vi "New Image (ARGB Array).vi"(7 "Set Alpha Values to 255 (Default: True)":bool=TRUE, 8 "error in (no error)":errorcluster, 11 "U32 ARBG Data":u32[][](array[numeric])) -> (0 "error out":errorcluster, 3 "ARGB Image":T1)   [LabVIEW 2020, in "image.lvlib"]
doc: "Create a New Image. The New Image data can be prep-populated with the given array of U32 image data.\n\nTo create a New Image which has a preallocated size with a uniform colour, use the \"New Image (ARGB Preallocated).vi\""
uses:
  image.lvlib
  ARGB Image.ctl
  common/common.lvlib
  common/bin/gartoolkit_32-1.dll
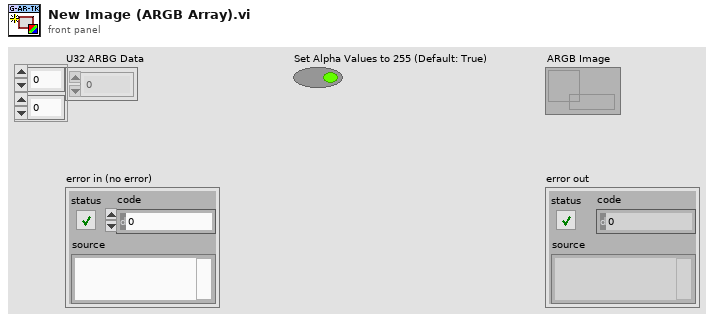
[diagram p1: front panel]
types:
  T1 = typedef "image.lvlib/ARGB Image.ctl" = refnum<data-value>
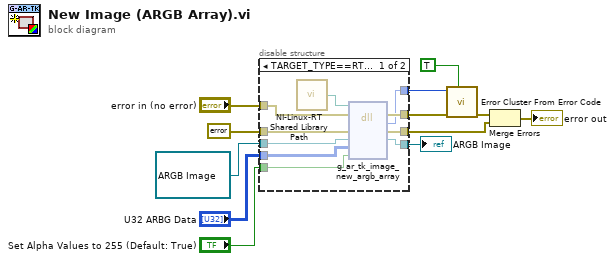
[diagram p0: block diagram]
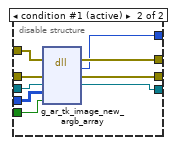
[diagram p2: hidden frame]
diagram:
  n1 = disable-structure shown="TARGET_TYPE==RT&&OS==Linux" {
    disable-tunnel: "error in (no error)" -> [w22 w31]
    disable-tunnel: errorcluster {"status"=FALSE, "code"=0, "source"=""} ("error constant") -> [w21 w30]
    disable-tunnel: T1 refnum ("ARGB Image") -> [w20 w29]
    disable-tunnel: "U32 ARBG Data" -> [w19 w28]
    disable-tunnel: "Set Alpha Values to 255 (Default: True)" -> [w18 w27]
    disable-tunnel: [w17 w26] -> w5
    disable-tunnel: [w16 w25] -> w4
    disable-tunnel: [w15 w24] -> w3
    disable-tunnel: [w14 w23] -> w2
    frame condition #0 {
      n2 = call "NI-Linux-RT Shared Library Path.vi"() -> ("Path"=w13:path)
      n3 = dll-call lib="?" fn="g_ar_tk_image_new_argb_array" ("g_ar_toolkit.*.*:g_ar_tk_image_create")(path in=w13, error in=w22, "error_cluster"=w21, "EDVR"=w20, "array_handle"=w19, "set_alpha_channel_to_255"=w18) -> (error out=w17:errorcluster, w16:i32, "error_cluster"=w15:errorcluster, "EDVR"=w14:T1)  [unwired: 3 in, 1 out]
    }
    frame condition #1 (active) {
      n4 = dll-call lib="C:/serenial/lib/g-augmented-reality-toolkit/LabVIEW/common/bin/gartoolkit_*-1.*" fn="g_ar_tk_image_new_argb_array" ("g_ar_toolkit.*.*:g_ar_tk_image_create")(error in=w31, "error_cluster"=w30, "EDVR"=w29, "array_handle"=w28, "set_alpha_channel_to_255"=w27) -> (error out=w26:errorcluster, w25:i32, "error_cluster"=w24:errorcluster, "EDVR"=w23:T1)  [unwired: 4 in, 1 out]
    }
  }
  "ARGB Image" <- w2
  n5 = call <vilib>:"Error Cluster From Error Code.vi"("show call chain? (False)"=TRUE, "error in (no error)"=w5, "error code (0)"=w4) -> ("error out"=w11:errorcluster)  [unwired: 6 in]
  n6 = Merge Errors(w11, w3) -> (→"error out":errorcluster)
